vi "cRIO HOST_Simulation.vi"(11 "MeasSet":T1={"Data Rate 9775"=3.0, "Data Rate 9215"=1200000.0, "Samples RMS 9215"=480000, "Samples RMS 9775"=3}) -> (1 "current time":timestamp, 2 "9775":dbl[](array[numeric]), 3 "9215":dbl[](array[numeric]))   [LabVIEW 2019, in "DAQ_Engine.lvclass"]
uses:
  DAQ_Engine.lvclass
  Common/DataTypes/Measurement Config--cluster.ctl
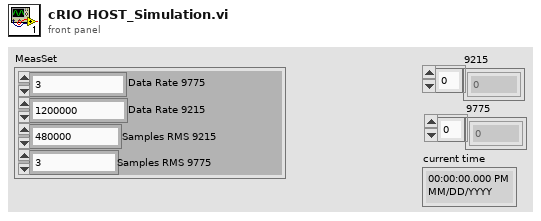
[diagram p1: front panel]
types:
  T1 = typedef "Measurement Config--cluster.ctl" = cluster{"Data Rate 9775":dbl, "Data Rate 9215":dbl, "Samples RMS 9215":u32, "Samples RMS 9775":u32}
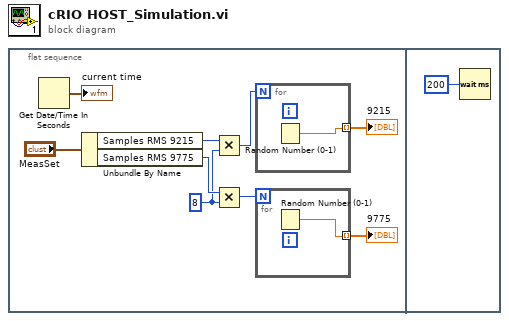
[diagram p0: block diagram]
diagram:
  n1 = flat-sequence {
    frame #0 {
      w1 = u32 8 ("y")
      n2 = Get Date/Time In Seconds() -> (seconds since 1Jan1904=→"current time":timestamp)
      n3 = Unbundle By Name("MeasSet") -> ("Samples RMS 9215"=w8:u32, "Samples RMS 9775"=w7:u32)
      n4 = Multiply(x=w8, y=w1) -> (x*y=w3:u32)
      n5 = Multiply(x=w7, y=w1) -> (x*y=w2:u32)
      n6 = for {
        N: w3 -> [_]
        tunnel: [w11] -> w6 mode=indexing
        n7 = Random Number (0-1)() -> (number: 0 to 1=w11:dbl)
      }
      "9215" <- w6
      n8 = for {
        N: w2 -> [_]
        tunnel: [w10] -> w5 mode=indexing
        n9 = Random Number (0-1)() -> (number: 0 to 1=w10:dbl)
      }
      "9775" <- w5
    }
    frame #1 {
      n10 = Wait (ms)(milliseconds to wait=u32 200) -> ()  [unwired: 1 out]
    }
  }
